vi "Subscribe (async) JSON.vi"(7 "Options":string, 8 "error in (no error)":errorcluster, 9 "Topic":string, 11 "WAMP Client in":refnum<class "WAMP Client.lvclass">) -> (0 "error out":errorcluster, 2 "notifier out":refnum<notifier>, 3 "WAMP Client out":refnum<class "WAMP Client.lvclass">)   [LabVIEW 2020, in "wamplv.lvlib" / "WAMP Client.lvclass"]
uses:
  WAMP Client.lvclass
  WAMP Client.lvclass/WAMP Client.ctl
  Private/Requests/Subscribe/Subscribe JSON/Subscribe JSON.lvclass
  C:/local/wamplv/Private/Requests/IGenericWithOutputInternalMessage/IGenericWithOutputInternalMessage/IGenericWithOutputInternalMessage.lvclass
  C:/local/wamplv/Private/Requests/IInternalMessage/IInternalMessage.lvclass
  C:/local/wamplv/Private/Requests/Subscribe/ISubscribe/ISubscribe.lvclass
  C:/local/wamplv/Private/Requests/IContainersNotiferOrEvents/IContainersNotiferOrEvents.lvclass
  C:/local/wamplv/Private/Requests/Subscribe/Subscribe JSON/Subscribe JSON.lvclass
  Private/Requests/Subscribe/Subscribe result (JSON).ctl
  wamplv.lvlib
  Private/Message loop classes/Subscription details/SubscriptionDetails JSON/SubscriptionDetails JSON.lvclass
  Private/Message loop classes/ErrorOrSuccess JSON/ErrorOrSuccess JSON.lvclass
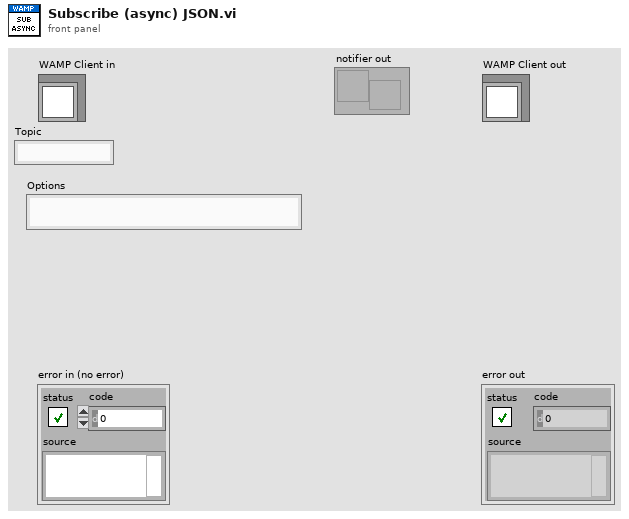
[diagram p1: front panel]
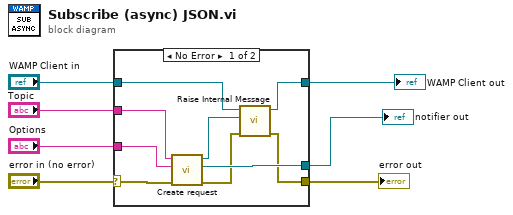
[diagram p0: block diagram]
diagram:
  n1 = case shown="No Error" "error in (no error)" {
    selector: "error in (no error)" -> [w16 w18]
    tunnel: [w11 w18] -> w6
    tunnel: [w9 w17] -> w4
    tunnel: "WAMP Client in" -> [w10 w17]
    tunnel: "Topic" -> [w14 _]
    tunnel: [w13 _] -> w2
    tunnel: "Options" -> [w15 _]
    frame No Error {
      n2 = call "Create request.vi"("error in (no error)"=w16, "Options"=w15, "Topic"=w14) -> ("error out"=w12:errorcluster, "notifier out"=w13:refnum<notifier>, "Subscribe JSON out"=w8:refnum<class "Subscribe JSON.lvclass">)  [unwired: 6 in]
      n3 = call "Raise Internal Message.vi"("error in (no error)"=w12, "IInternalMessage"=w8, "WAMP Client in"=w10) -> ("error out"=w11:errorcluster, "WAMP Client out"=w9:refnum<class "WAMP Client.lvclass">)  [unwired: 7 in]
    }
    frame Error {
    }
  }
  "error out" <- w6
  "WAMP Client out" <- w4
  "notifier out" <- w2
